vi "Write Initial Data from Cluster.vi"(1 "Correlator Initial Data":T1={"Max Exposition Time (ms)"=1, "Channel1 Threshold Voltage (mV)"=1, "Channel1 Pulse Front"="", "Channel2 Threshold Voltage (mV)"=1, "Channel2 Pulse Front"="", "Channel3 Threshold Voltage (mV)"=1, "Channel3 Pulse Front "="", "Channel4 Threshold Voltage (mV)"=1, "Channel4 Pulse Front "="", "Single Count Enable"={"Channel1"=FALSE, "Channel2"=FALSE, "Channel3"=FALSE, "Channel4"=FALSE}, "Single Count Max"=1, "Sum Count Enable"={"Channel1"=FALSE, "Channel2"=FALSE, "Channel3"=FALSE, "Channel4"=FALSE}, "Sum Count Max"=1, "Start-Stop1 Multyplex"={"Stop Channel"="", "Start Channel"=""}, "Stop Delay 1 (ns)"=1, "Window Length 1 (ns)"=4, "Window Offset 1 (ns) "=4, "Conditional Correlation 1"="", "Histogram Bin 1"="", "Histogram Start 1 (ns) "=4, "Start-Stop2 Multyplex "={"Stop Channel"="", "Start Channel"=""}, "Stop Delay 2 (ns)"=1, "Window Length 2 (ns) "=4, "Window Offset 2 (ns) "=4, "Conditional Correlation 2"="", "Histogram Bin 2"="", "Histogram Start 2 (ns)  "=4, "Start-Stop3 Multyplex"={"Stop Channel"="", "Start Channel"=""}, "Stop Delay 3 (ns)"=1, "Window Length 3 (ns) "=4, "Window Offset 3 (ns) "=4, "Conditional Correlation 3"="", "Histogram Bin 3"="", "Histogram Start 3 (ns) "=4, "Start-Stop4 Multyplex"={"Stop Channel"="", "Start Channel"=""}, "Stop Delay 4 (ns)"=1, "Window Length 4 (ns)  "=4, "Window Offset 4 (ns) "=4, "Conditional Correlation 4"="", "Histogram Bin 4"="", "Histogram Start 4 (ns)  "=4, "Coincidence Count Enable"={"Start-Stop1"=FALSE, "Start-Stop2"=FALSE, "Start-Stop3"=FALSE, "Start-Stop4"=FALSE}, "Coincidence Count Max"=1, "Coincidence Sum Enable 2"={"Start-Stop1"=FALSE, "Start-Stop2"=FALSE, "Start-Stop3"=FALSE, "Start-Stop4"=FALSE}, "Coincidence Sum Max"=1, "Output Channel Enable"={"Channel1"=FALSE, "Channel2"=FALSE, "Channel3"=FALSE, "Channel4"=FALSE}, "Output Channel Inversion"={"Channel1"=FALSE, "Channel2"=FALSE, "Channel3"=FALSE, "Channel4"=FALSE, "Output"=FALSE}} {"Coincidence Sum Max" min=1 max=16777215 step=1 format="%.7e"; "Coincidence Count Max" min=1 max=16777215 step=1 format="%.7e"; "Histogram Start 4 (ns)" min=0 max=120000 step=2; "Window Offset 4 (ns)" min=0 max=120000 step=2; "Window Length 4 (ns)" min=4 max=60000 step=4; "Stop Delay 4 (ns)" min=0 max=1008 step=16; "Histogram Start 3 (ns)" min=0 max=120000 step=2; "Window Offset 3 (ns)" min=0 max=120000 step=2; "Window Length 3 (ns)" min=4 max=60000 step=4; "Stop Delay 3 (ns)" min=0 max=1008 step=16; "Histogram Start 2 (ns)" min=0 max=120000 step=2; "Window Offset 2 (ns)" min=0 max=120000 step=2; "Window Length 2 (ns)" min=4 max=60000 step=4; "Stop Delay 2 (ns)" min=0 max=1008 step=16; "Histogram Start 1 (ns)" min=0 max=120000 step=2; "Window Offset 1 (ns)" min=0 max=120000 step=2; "Window Length 1 (ns)" min=4 max=60000 step=4; "Stop Delay 1 (ns)" min=0 max=1008 step=16; "Sum Count Max" min=1 max=16777215 step=1 format="%.7e"; "Single Count Max" min=1 max=16777215 step=1 format="%.7e"; "Channel4 Threshold Voltage (mV)" min=0 max=5000 step=10; "Channel3 Threshold Voltage (mV)" min=0 max=5000 step=10; "Channel2 Threshold Voltage (mV)" min=0 max=5000 step=10; "Channel1 Threshold Voltage (mV)" min=0 max=5000 step=10; "Max Exposition Time (ms)" min=1 max=3600000000 step=1 format="%.9e"}) -> (0 "Write OK":bool)   [LabVIEW 2012]
panel:
  out "string":string
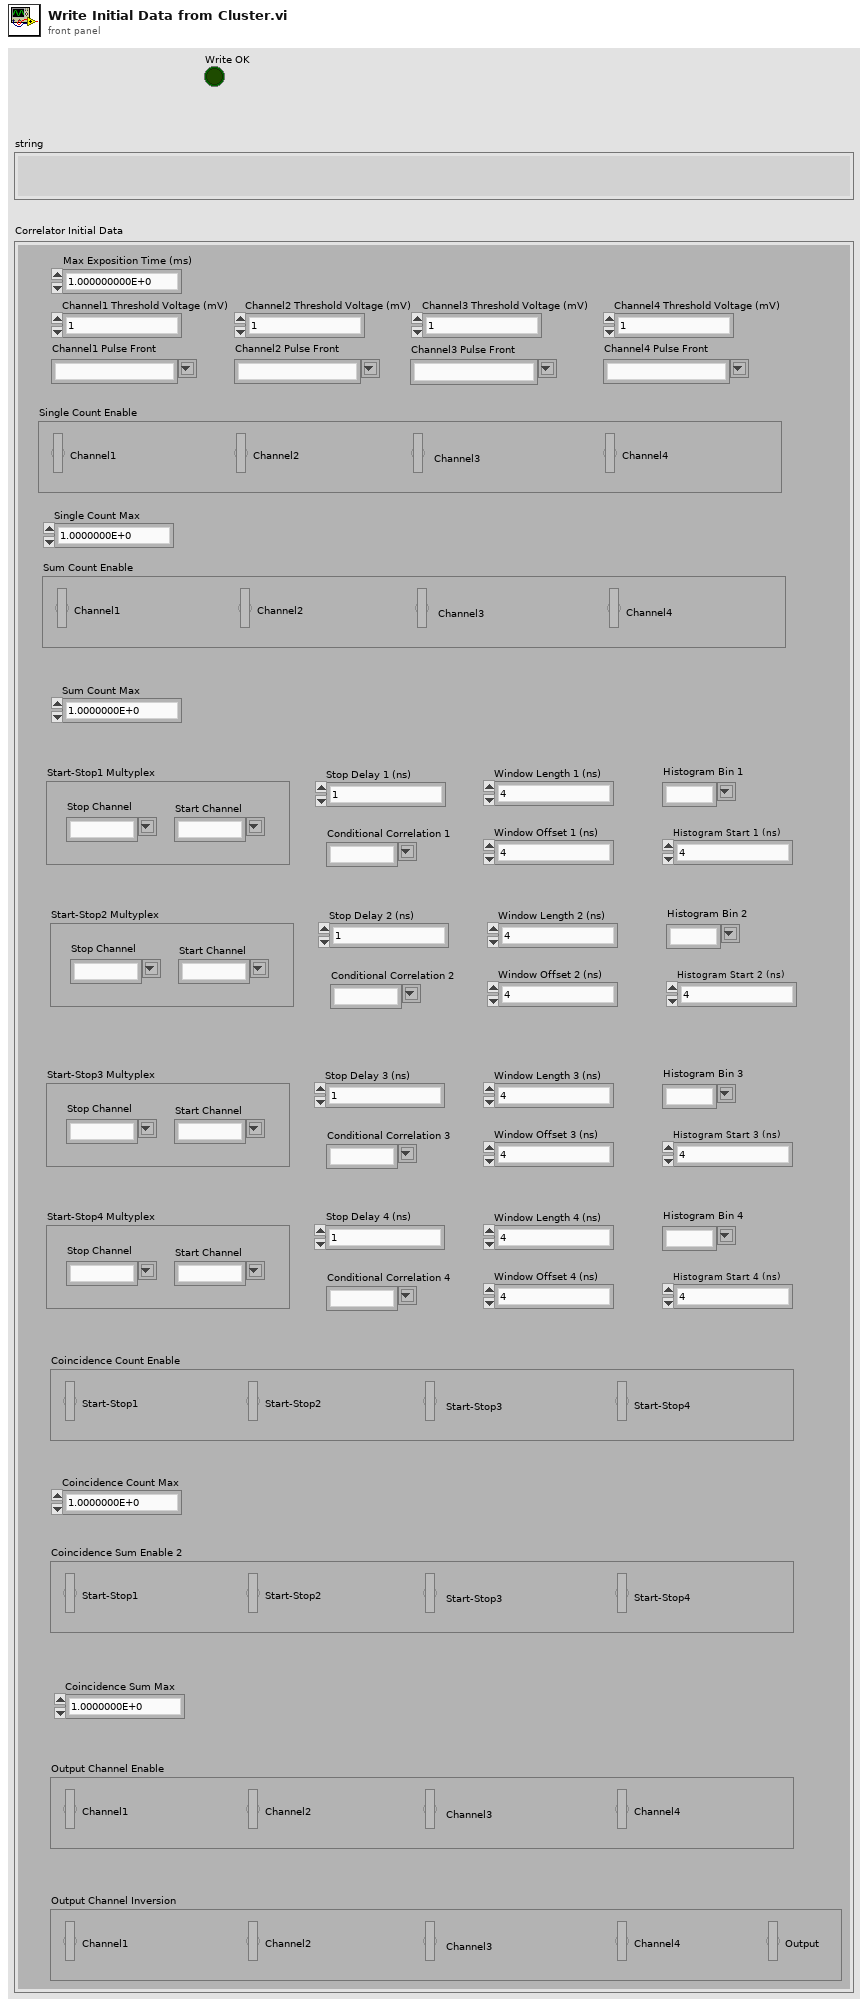
[diagram p1: front panel]
types:
  T1 = cluster{"Max Exposition Time (ms)":i64, "Channel1 Threshold Voltage (mV)":i32, "Channel1 Pulse Front":string, "Channel2 Threshold Voltage (mV)":i32, "Channel2 Pulse Front":string, "Channel3 Threshold Voltage (mV)":i32, "Channel3 Pulse Front ":string, "Channel4 Threshold Voltage (mV)":i32, "Channel4 Pulse Front ":string, "Single Count Enable":cluster{"Channel1":bool, "Channel2":bool, "Channel3":bool, "Channel4":bool}, "Single Count Max":i32, "Sum Count Enable":cluster{"Channel1":bool, "Channel2":bool, "Channel3":bool, "Channel4":bool}, "Sum Count Max":i32, "Start-Stop1 Multyplex":cluster{"Stop Channel":string, "Start Channel":string}, "Stop Delay 1 (ns)":i16, "Window Length 1 (ns)":i32, "Window Offset 1 (ns) ":i32, "Conditional Correlation 1":string, "Histogram Bin 1":string, "Histogram Start 1 (ns) ":i32, "Start-Stop2 Multyplex ":cluster{"Stop Channel":string, "Start Channel":string}, "Stop Delay 2 (ns)":i16, "Window Length 2 (ns) ":i32, "Window Offset 2 (ns) ":i32, "Conditional Correlation 2":string, "Histogram Bin 2":string, "Histogram Start 2 (ns)  ":i32, "Start-Stop3 Multyplex":cluster{"Stop Channel":string, "Start Channel":string}, "Stop Delay 3 (ns)":i16, "Window Length 3 (ns) ":i32, "Window Offset 3 (ns) ":i32, "Conditional Correlation 3":string, "Histogram Bin 3":string, "Histogram Start 3 (ns) ":i32, "Start-Stop4 Multyplex":cluster{"Stop Channel":string, "Start Channel":string}, "Stop Delay 4 (ns)":i16, "Window Length 4 (ns)  ":i32, "Window Offset 4 (ns) ":i32, "Conditional Correlation 4":string, "Histogram Bin 4":string, "Histogram Start 4 (ns)  ":i32, "Coincidence Count Enable":cluster{"Start-Stop1":bool, "Start-Stop2":bool, "Start-Stop3":bool, "Start-Stop4":bool}, "Coincidence Count Max":i32, "Coincidence Sum Enable 2":cluster{"Start-Stop1":bool, "Start-Stop2":bool, "Start-Stop3":bool, "Start-Stop4":bool}, "Coincidence Sum Max":i32, "Output Channel Enable":cluster{"Channel1":bool, "Channel2":bool, "Channel3":bool, "Channel4":bool}, "Output Channel Inversion":cluster{"Channel1":bool, "Channel2":bool, "Channel3":bool, "Channel4":bool, "Output":bool}}
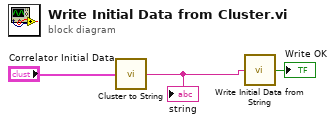
[diagram p0: block diagram]
diagram:
  n1 = call "Cluster to String.vi"("Correlator Initial Data"="Correlator Initial Data") -> ("string"=w2:string)
  "string" <- w2
  n2 = call "Write Initial Data from String.vi"("Data"=w2) -> ("Write OK"=→"Write OK":bool)
